vi "Newmark-Test.vi"() -> ()   [LabVIEW 2011]
panel:
  in  "Auto-Catch":bool
  in  "Pre":string
  in  "Post":string
  out "FoyerSonde":i32
  in  "Foyer":i32=5000
  in  "go Sud":bool caption="Ajustement Sud"
  in  "go Ouest":bool caption="Ajustement Est"
  in  "go Nord":bool caption="Ajustement Nord"
  in  "go Est":bool caption="Ajustement Ouest"
  in  "enfoncé":bool
  in  "Foyer+":bool caption="Foyer +"
  in  "Foyer-":bool caption="Foyer -"
  out "X Home":dbl
  in  "Accel":dbl=25000.0
  in  "Fast":dbl=25000.0
  in  "Slow":dbl=10.0
  in  "ActiveStages":string[](array[string])=["AX"]
  out "T Axis":dbl
  out "Z Axis":dbl
  out "Y Axis":dbl
  out "X Axis":dbl
  in  "Auto-Query":bool
  out "In use ?":bool
  in  "CLEAR":bool
  in  "stop":bool
  out "Communication Log":string
  in  "Command String":string
  in  "SendChar":bool
  in  "SendPredefined":bool
  in  "Predefined Commmands":i32(ring) items=["Stop All [SA]", "Referencement", "Home [HM]", "Home Reverse [HR]", "Report Position [PE]", "Status All"]
  in  "Timeout":u32=10000
  in  "baud rate":u32=9600
  in  "VISA resource name":refnum<visa-resource-name>="COM10"
  # "Z"
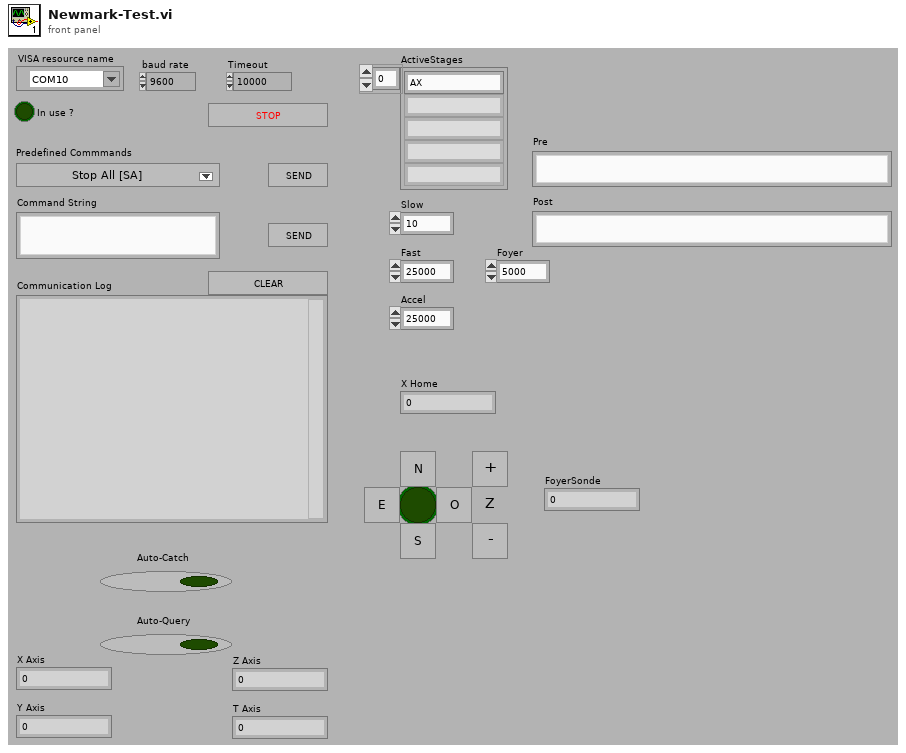
[diagram p1: front panel]
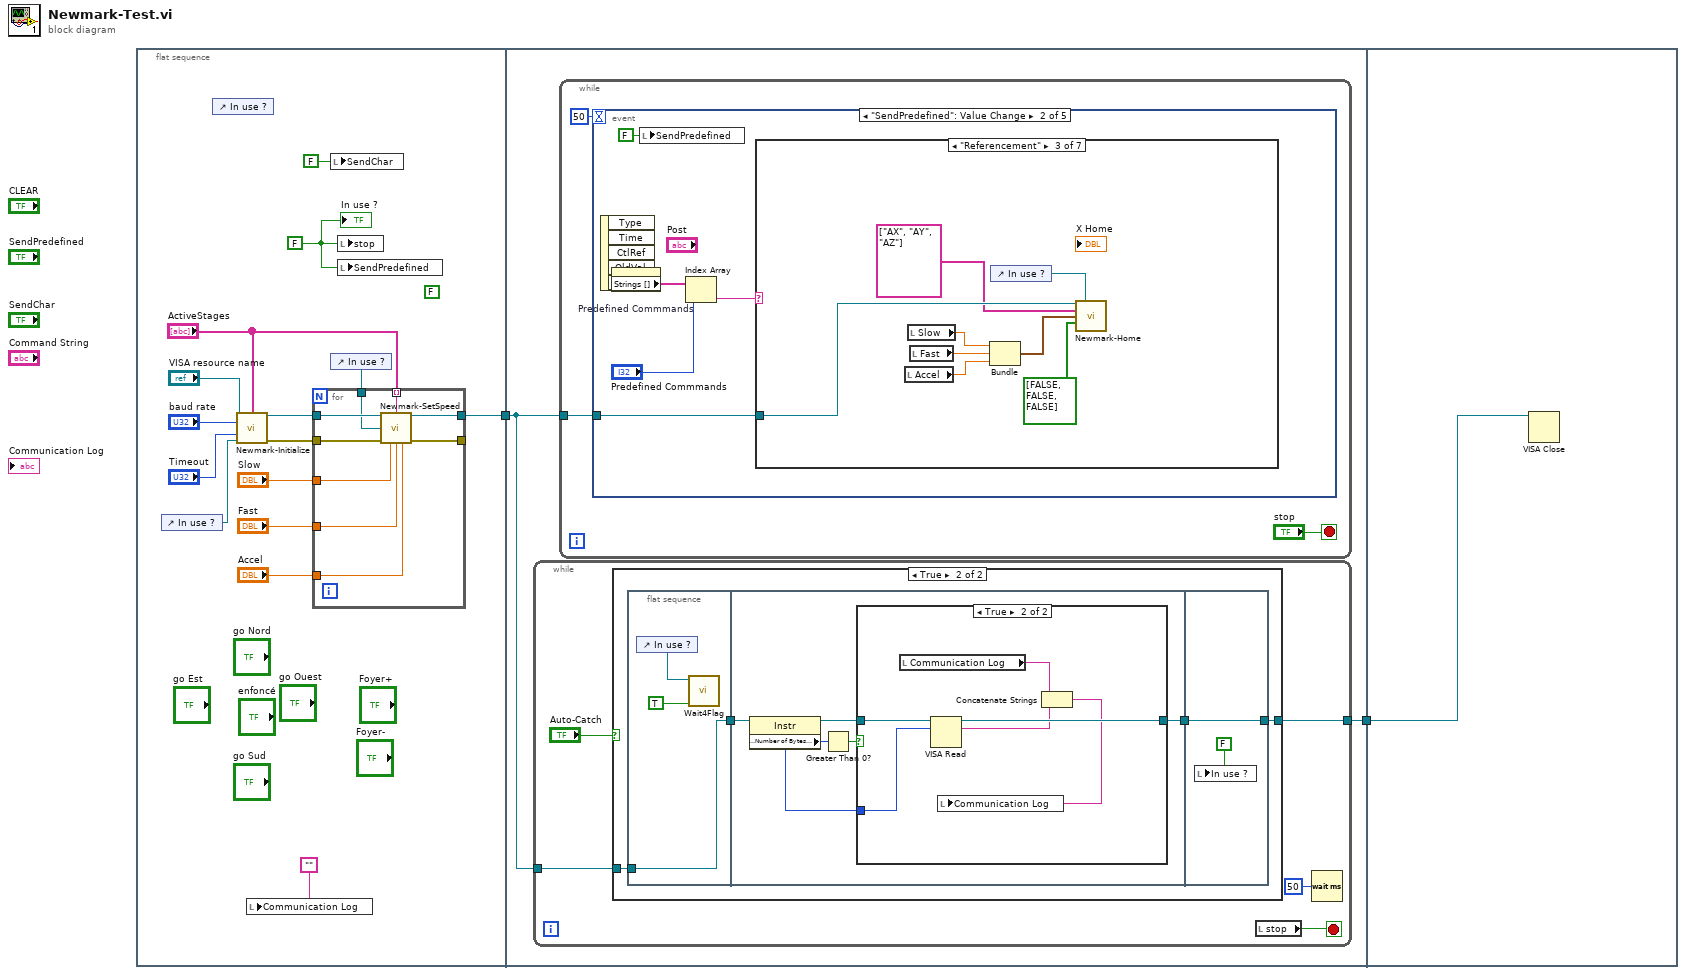
[diagram p0: block diagram]
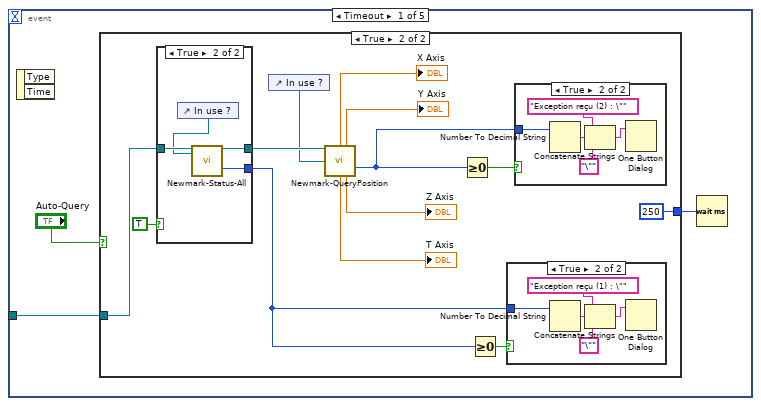
[diagram p4: hidden frame]
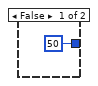
[diagram p5: hidden frame]
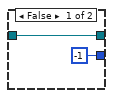
[diagram p6: hidden frame]
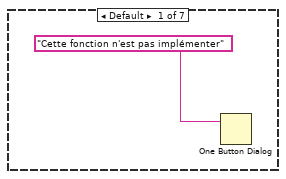
[diagram p9: hidden frame]
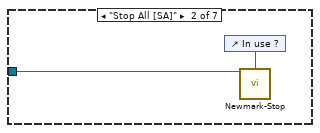
[diagram p10: hidden frame]
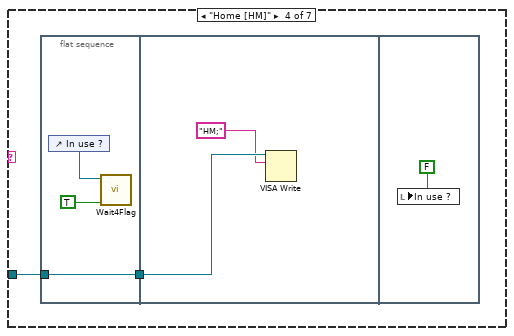
[diagram p11: hidden frame]
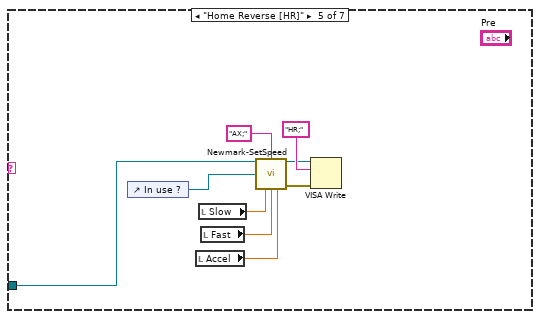
[diagram p12: hidden frame]
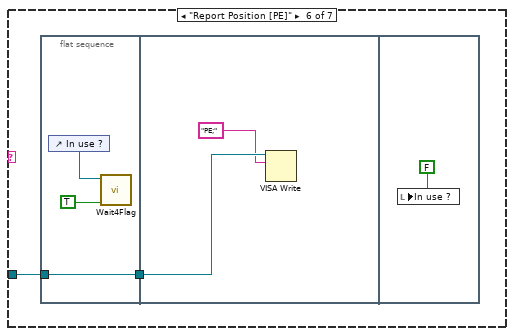
[diagram p13: hidden frame]
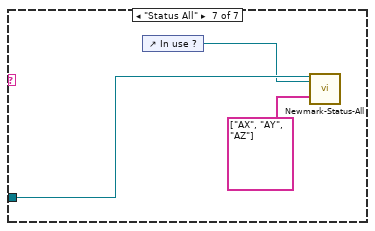
[diagram p14: hidden frame]
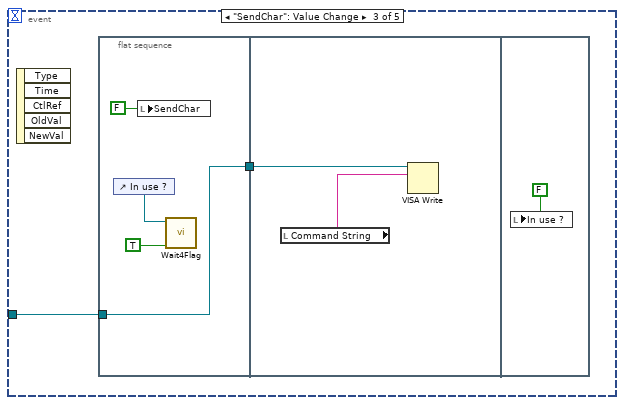
[diagram p15: hidden frame]
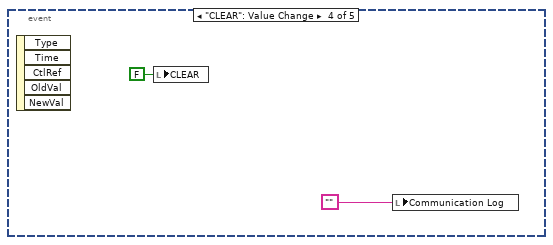
[diagram p16: hidden frame]
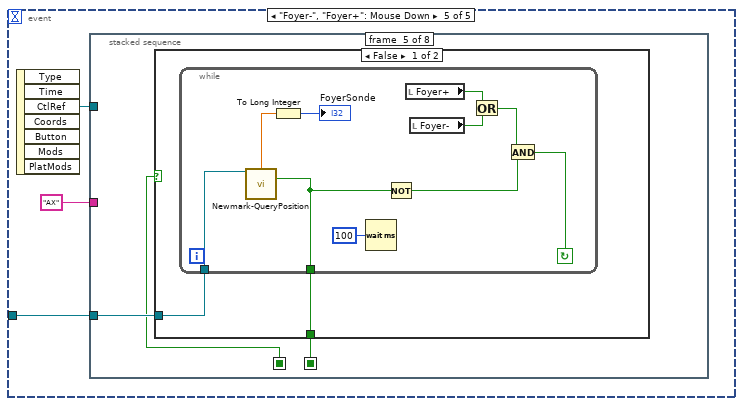
[diagram p17: hidden frame]
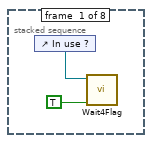
[diagram p18: hidden frame]
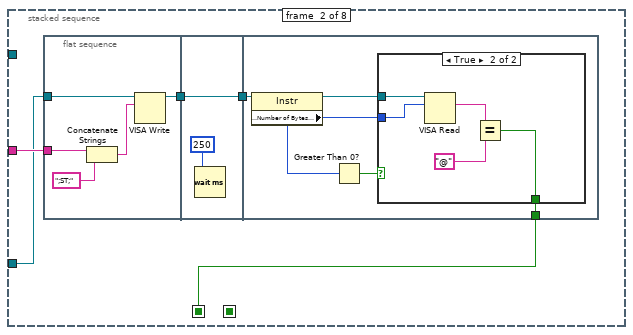
[diagram p19: hidden frame]
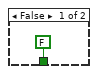
[diagram p20: hidden frame]
diagram:
  n1 = flat-sequence {
    tunnel: [w11] -> w1
    tunnel: [w27] -> w2
    tunnel: w1 -> [w28]
    tunnel: w2 -> [w236]
    frame #0 {
      w16 = FALSE ("Enable Termination\nChar (T)")
      (unwired) FALSE ("Enable Termination\nChar (T)")
      n2 = control-ref of="In use ?"() -> (w3:refnum<vi>)
      n3 = control-ref of="In use ?"() -> ()  [unwired: 1 out]
      n4 = call "Newmark-Initialize.vi"("VISA resource name"="VISA resource name", "ActiveStages"="ActiveStages", "baud rate"="baud rate", "Timeout"="Timeout", "Bool Refnum"=w3) -> ("VISA resource name out"=w10:refnum<visa-resource-name>, "Error OUT"=w8:errorcluster)  [unwired: 8 in, 1 out]
      n5 = local write "Communication Log"("") -> ()
      n6 = local write "SendChar"(FALSE ("Enable Termination\nChar (T)")) -> ()
      n7 = control-ref of="In use ?"() -> (w4:refnum<vi>)
      n8 = for {
        tunnel: w10 -> [w26]
        tunnel: [w25] -> w11
        tunnel: "ActiveStages" -> [w24] mode=indexing
        tunnel: w8 -> [w23]
        tunnel: [w22] -> _
        tunnel: "Slow" -> [w21]
        tunnel: "Fast" -> [w20]
        tunnel: "Accel" -> [w19]
        tunnel: w4 -> [w18]
        n9 = call "Newmark-SetSpeed.vi"("Table VRN"=w26, "StageTAG"=w24, "Bool Refnum"=w18, "Error IN"=w23, "Vitesse Lente"=w21, "Vitesse Rapide"=w20, "Accélération"=w19) -> ("Table VRN OUT"=w25:refnum<visa-resource-name>, "Error OUT"=w22:errorcluster)  [unwired: 6 in, 1 out]
      }
      n10 = local write "stop"(w16) -> ()
      n11 = local write "SendPredefined"(w16) -> ()
      "In use ?" <- w16
    }
    frame #1 {
      n12 = while {
        tunnel: w28 -> [w32]
        tunnel: [w31] -> w27
        stop <- w33 stop-if-true
        n13 = case shown="True" "Auto-Catch" {
          tunnel: w32 -> [w34 w36]
          tunnel: [w34 w35] -> w31
          frame False {
          }
          frame True {
            n14 = flat-sequence {
              tunnel: w36 -> [w41]
              tunnel: [w41] -> w38
              tunnel: w38 -> [w46]
              tunnel: [w43] -> w37
              tunnel: [w55] -> w35
              tunnel: w37 -> [w55]
              frame #0 {
                n15 = control-ref of="In use ?"() -> (w40:refnum<vi>)
                n16 = call "Wait4Flag.vi"("Raise Flag ?"=TRUE, "Ctl Refnum IN"=w40) -> ()  [unwired: 8 in, 2 out]
              }
              frame #1 {
                n17 = property class="Instr"(reference=w46) -> (reference out=w44:refnum<visa-resource-name>, "Serial Settings:Number of Bytes at Serial Port"=w42:u32)  [unwired: 1 in, 1 out]
                n18 = Greater Than 0?(x=w42) -> (x > 0?=w45:bool)
                n19 = case shown="True" w45 {
                  tunnel: w44 -> [w47 w53]
                  tunnel: [w47 w51] -> w43
                  tunnel: w42 -> [_ w52]
                  frame False {
                  }
                  frame True {
                    n20 = local read "Communication Log"() -> (w49:string)
                    n21 = VISA Read(VISA resource name=w53, byte count=w52) -> (VISA resource name out=w51:refnum<visa-resource-name>, read buffer=w50:string)  [unwired: 1 in, 2 out]
                    n22 = Concatenate Strings(w49, w50) -> (w48:string)
                    n23 = local write "Communication Log"(w48) -> ()
                  }
                }
              }
              frame #2 {
                n24 = local write "In use ?"(FALSE ("Enable Termination\nChar (T)")) -> ()
              }
            }
          }
        }
        n25 = local read "stop"() -> (w33:bool)
        n26 = Wait (ms)(milliseconds to wait=u32 50) -> ()  [unwired: 1 out]
      }
      n27 = while {
        tunnel: w28 -> [w57]
        stop <- "stop" stop-if-true
        n28 = event shown="[1] \"SendPredefined\": Value Change" {
          selector: _ -> [_ _ _ _ _]
          dyn-events: _ -> [_ _ _ _ _]
          timeout: 50 -> [_ _ _ _ _]
          tunnel: w57 -> [w61 w92 w137 _ w149]
          event Timeout {
            n29 = event-data() -> ()  [unwired: 1 in, 2 out]
            n30 = case shown="True" "Auto-Query" {
              tunnel: w61 -> [_ w67]
              tunnel: [u32 50 u32 250] -> w59
              frame False {
              }
              frame True {
                n31 = case shown="True" TRUE {
                  tunnel: w67 -> [w77 w81]
                  tunnel: [w77 w80] -> w66
                  tunnel: [-1 ("Exception") w79] -> w65
                  frame False {
                  }
                  frame True {
                    n32 = control-ref of="In use ?"() -> (w78:refnum<vi>)
                    n33 = call "Newmark-Status-All.vi"("Table VRN IN"=w81, "Bool Refnum"=w78) -> ("Table VRN OUT"=w80:refnum<visa-resource-name>, "Exception"=w79:i32)  [unwired: 5 in, 11 out]
                  }
                }
                n34 = control-ref of="In use ?"() -> (w63:refnum<vi>)
                n35 = call "Newmark-QueryPosition.vi"("Table VRN IN"=w66, "Bool Refnum"=w63) -> ("X Axis"=→"X Axis":dbl, "Y Axis"=→"Y Axis":dbl, "Exception"=w71:i32, "T Axis"=→"T Axis":dbl, "Z Axis"=→"Z Axis":dbl)  [unwired: 6 in, 3 out]
                n36 = Greater Or Equal To 0?(x=w71) -> (x >= 0?=w70:bool)
                n37 = Greater Or Equal To 0?(x=w65) -> (x >= 0?=w69:bool)
                n38 = case shown="True" w69 {
                  tunnel: w65 -> [_ w83]
                  frame False {
                  }
                  frame True {
                    n39 = Number To Decimal String(number=w83) -> (decimal integer string=w84:string)  [unwired: 1 in]
                    n40 = Concatenate Strings("Exception reçu (1) : \"" ("string"), w84, "\"" ("string")) -> (w82:string)
                    n41 = One Button Dialog(message=w82) -> ()  [unwired: 1 in, 1 out]
                  }
                }
                n42 = case shown="True" w70 {
                  tunnel: w71 -> [_ w88]
                  frame False {
                  }
                  frame True {
                    n43 = Number To Decimal String(number=w88) -> (decimal integer string=w89:string)  [unwired: 1 in]
                    n44 = Concatenate Strings("Exception reçu (2) : \"" ("string"), w89, "\"" ("string")) -> (w87:string)
                    n45 = One Button Dialog(message=w87) -> ()  [unwired: 1 in, 1 out]
                  }
                }
              }
            }
            n46 = Wait (ms)(milliseconds to wait=w59) -> ()  [unwired: 1 out]
          }
          event "SendPredefined": Value Change {
            n47 = event-data() -> ()  [unwired: 1 in, 5 out]
            n48 = property on="Predefined Commmands" class="Ring (strict)"() -> ("Strings []"=w96:string[])  [unwired: 2 in, 2 out]
            n49 = local write "SendPredefined"(FALSE ("SendPredefined")) -> ()
            n50 = Index Array(array=w96, index="Predefined Commmands") -> (element=w94:string)
            n51 = case shown="\"Referencement\"" w94 {
              tunnel: w92 -> [_ w99 w107 w109 w116 w126 w135]
              frame Default {
                n52 = One Button Dialog(message="Cette fonction n'est pas implémenter") -> ()  [unwired: 1 in, 1 out]
              }
              frame "Stop All [SA]" {
                n53 = control-ref of="In use ?"() -> (w98:refnum<vi>)
                n54 = call "Newmark-Stop.vi"("Table VRN IN"=w99, "Bool Refnum"=w98) -> ()  [unwired: 12 in, 2 out]
              }
              frame "Referencement" {
                n55 = local read "Accel"() -> (w102:dbl)
                n56 = local read "Slow"() -> (w104:dbl)
                n57 = local read "Fast"() -> (w103:dbl)
                n58 = Bundle("Slow"=w104, "Fast"=w103, "Accel"=w102) -> (w101:cluster{"Slow":dbl, "Fast":dbl, "Accel":dbl})  [unwired: 1 in]
                n59 = control-ref of="In use ?"() -> (w100:refnum<vi>)
                n60 = call "Newmark-Home.vi"("Table VRN IN"=w107, "Comm Active"=w100, "StageTAGs"=string[] ["AX", "AY", "AZ"], "Velocities"=w101, "HomeReverse?"=bool[] [FALSE, FALSE, FALSE]) -> ()  [unwired: 9 in, 2 out]
              }
              frame "Home [HM]" {
                n61 = flat-sequence {
                  tunnel: w109 -> [w110]
                  tunnel: [w110] -> w108
                  tunnel: w108 -> [w114]
                  frame #0 {
                    n62 = control-ref of="In use ?"() -> (w111:refnum<vi>)
                    n63 = call "Wait4Flag.vi"("Raise Flag ?"=TRUE, "Ctl Refnum IN"=w111) -> ()  [unwired: 8 in, 2 out]
                  }
                  frame #1 {
                    n64 = VISA Write(VISA resource name=w114, write buffer="HM;") -> ()  [unwired: 1 in, 3 out]
                  }
                  frame #2 {
                    n65 = local write "In use ?"(FALSE ("Enable Termination\nChar (T)")) -> ()
                  }
                }
              }
              frame "Home Reverse [HR]" {
                n66 = control-ref of="In use ?"() -> (w117:refnum<vi>)
                n67 = local read "Accel"() -> (w118:dbl)
                n68 = local read "Slow"() -> (w120:dbl)
                n69 = local read "Fast"() -> (w119:dbl)
                n70 = call "Newmark-SetSpeed.vi"("Table VRN"=w116, "StageTAG"="AX;", "Bool Refnum"=w117, "Vitesse Lente"=w120, "Vitesse Rapide"=w119, "Accélération"=w118) -> ("Table VRN OUT"=w123:refnum<visa-resource-name>, "Error OUT"=w122:errorcluster)  [unwired: 7 in, 1 out]
                n71 = VISA Write(VISA resource name=w123, write buffer="HR;", error in (no error)=w122) -> ()  [unwired: 3 out]
              }
              frame "Report Position [PE]" {
                n72 = flat-sequence {
                  tunnel: w126 -> [w127]
                  tunnel: [w127] -> w125
                  tunnel: w125 -> [w131]
                  frame #0 {
                    n73 = control-ref of="In use ?"() -> (w128:refnum<vi>)
                    n74 = call "Wait4Flag.vi"("Raise Flag ?"=TRUE, "Ctl Refnum IN"=w128) -> ()  [unwired: 8 in, 2 out]
                  }
                  frame #1 {
                    n75 = VISA Write(VISA resource name=w131, write buffer="PE;") -> ()  [unwired: 1 in, 3 out]
                  }
                  frame #2 {
                    n76 = local write "In use ?"(FALSE ("Enable Termination\nChar (T)")) -> ()
                  }
                }
              }
              frame "Status All" {
                n77 = control-ref of="In use ?"() -> (w134:refnum<vi>)
                n78 = call "Newmark-Status-All.vi"("Table VRN IN"=w135, "Bool Refnum"=w134, "StageTag"=string[] ["AX", "AY", "AZ"]) -> ()  [unwired: 4 in, 13 out]
              }
            }
          }
          event "SendChar": Value Change {
            n79 = event-data() -> ()  [unwired: 1 in, 5 out]
            n80 = flat-sequence {
              tunnel: w137 -> [w139]
              tunnel: [w139] -> w136
              tunnel: w136 -> [w143]
              frame #0 {
                n81 = control-ref of="In use ?"() -> (w141:refnum<vi>)
                n82 = local write "SendChar"(FALSE ("Enable Termination\nChar (T)")) -> ()
                n83 = call "Wait4Flag.vi"("Raise Flag ?"=TRUE, "Ctl Refnum IN"=w141) -> ()  [unwired: 8 in, 2 out]
              }
              frame #1 {
                n84 = local read "Command String"() -> (w142:string)
                n85 = VISA Write(VISA resource name=w143, write buffer=w142) -> ()  [unwired: 1 in, 3 out]
              }
              frame #2 {
                n86 = local write "In use ?"(FALSE ("Enable Termination\nChar (T)")) -> ()
              }
            }
          }
          event "CLEAR": Value Change {
            n87 = event-data() -> ()  [unwired: 1 in, 5 out]
            n88 = local write "CLEAR"(FALSE ("CLEAR")) -> ()
            n89 = local write "Communication Log"("") -> ()
          }
          event "Foyer-", "Foyer+": Mouse Down {
            n90 = event-data() -> ("CtlRef"=w147:refnum<vi>)  [unwired: 1 in, 6 out]
            n91 = stacked-sequence {
              seq-local: [_ _ _ _ w200 _ _ _] -> [_ _ _ _ _ w216 _ _]
              seq-local: [_ w152 _ _ _ _ _ _] -> [_ _ w175 w182 w199 w215 w228 _]
              tunnel: w149 -> [_ w155 _ w184 w201 w218 _ _]
              tunnel: "AX" -> [_ w156 w176 w189 _ w217 w229 _]
              tunnel: w147 -> [_ _ _ w195 _ _ _ _]
              frame #0 {
                n92 = control-ref of="In use ?"() -> (w150:refnum<vi>)
                n93 = call "Wait4Flag.vi"("Raise Flag ?"=TRUE, "Ctl Refnum IN"=w150) -> ()  [unwired: 8 in, 2 out]
              }
              frame #1 {
                n94 = flat-sequence {
                  tunnel: w156 -> [w161]
                  tunnel: w155 -> [w158]
                  tunnel: [w157] -> w154
                  tunnel: w154 -> [w163]
                  tunnel: [w163] -> w153
                  tunnel: w153 -> [w168]
                  tunnel: [w164] -> w152
                  frame #0 {
                    n95 = Concatenate Strings(w161, ";ST;") -> (w159:string)
                    n96 = VISA Write(VISA resource name=w158, write buffer=w159) -> (VISA resource name out=w157:refnum<visa-resource-name>)  [unwired: 1 in, 2 out]
                  }
                  frame #1 {
                    n97 = Wait (ms)(milliseconds to wait=u32 250) -> ()  [unwired: 1 out]
                  }
                  frame #2 {
                    n98 = property class="Instr"(reference=w168) -> (reference out=w166:refnum<visa-resource-name>, "Serial Settings:Number of Bytes at Serial Port"=w165:u32)  [unwired: 1 in, 1 out]
                    n99 = Greater Than 0?(x=w165) -> (x > 0?=w167:bool)
                    n100 = case shown="True" w167 {
                      tunnel: w166 -> [_ w174]
                      tunnel: w165 -> [_ w173]
                      tunnel: [FALSE w170] -> w164
                      frame False {
                      }
                      frame True {
                        n101 = VISA Read(VISA resource name=w174, byte count=w173) -> (read buffer=w172:string)  [unwired: 1 in, 3 out]
                        n102 = Equal?(x=w172, y="@") -> (x = y?=w170:bool)
                      }
                    }
                  }
                }
              }
              frame #2 {
                # "Axe du foyer"
                n103 = case shown="False" w175 {
                  tunnel: w176 -> [w178 _]
                  frame False {
                    n104 = local read "Slow"() -> (w179:dbl)
                    n105 = local read "Accel"() -> (w177:dbl)
                    n106 = call "Newmark-SetSpeed.vi"("StageTAG"=w178, "Vitesse Lente"=w179, "Vitesse Rapide"="Foyer", "Accélération"=w177) -> ()  [unwired: 9 in, 3 out]
                  }
                  frame True {
                    n107 = One Button Dialog(message="L'étage du foyer a déjà atteint sa limte de déplacement.") -> ()  [unwired: 1 in, 1 out]
                  }
                }
              }
              frame #3 {
                n108 = property class="Bool (strict)"(reference=w195) -> ("Label.Text"=w194:string)  [unwired: 1 in, 2 out]
                n109 = local read "Foyer"() -> (w196:i32)
                n110 = Equal?(x=w194, y="Foyer+") -> (x = y?=w193:bool)
                n111 = Number To Decimal String(number=w196) -> (decimal integer string=w186:string)  [unwired: 1 in]
                n112 = Select(t="+", s=w193, f="-") -> (s? t:f=w187:string)
                n113 = Concatenate Strings(w189, ";JG", w187, w186, ";") -> (w183:string)
                n114 = case shown="False" w182 {
                  tunnel: w184 -> [w198 _]
                  tunnel: w183 -> [w197 _]
                  frame False {
                    n115 = VISA Write(VISA resource name=w198, write buffer=w197) -> ()  [unwired: 1 in, 3 out]
                  }
                  frame True {
                  }
                }
              }
              frame #4 {
                n116 = case shown="False" w199 {
                  tunnel: w201 -> [w203 _]
                  tunnel: [w202 FALSE ("OverTravel?")] -> w200
                  frame False {
                    n117 = while {
                      tunnel: w203 -> [w210]
                      tunnel: [w204] -> w202
                      stop <- w206 continue-if-true
                      n118 = call "Newmark-QueryPosition.vi"("Table VRN IN"=w210) -> ("X Axis"=w209:dbl, "Error?"=w204:bool)  [unwired: 7 in, 6 out]
                      n119 = To Long Integer(number=w209) -> (32bit integer=→"FoyerSonde":i32)
                      n120 = Wait (ms)(milliseconds to wait=u32 100) -> ()  [unwired: 1 out]
                      n121 = Not(x=w204) -> (.not. x?=w205:bool)
                      n122 = local read "Foyer+"() -> (w213:bool)
                      n123 = local read "Foyer-"() -> (w212:bool)
                      n124 = Or(x=w213, y=w212) -> (x .or. y?=w207:bool)
                      n125 = And(x=w207, y=w205) -> (x .and. y?=w206:bool)
                    }
                  }
                  frame True {
                  }
                }
              }
              frame #5 {
                n126 = case shown="True" w215 {
                  tunnel: w218 -> [w221 _]
                  tunnel: w217 -> [w220 _]
                  tunnel: w216 -> [w219 _]
                  frame False {
                    n127 = case shown="False" w219 {
                      tunnel: w221 -> [w225 _]
                      tunnel: w220 -> [w224 _]
                      frame False {
                        n128 = Concatenate Strings(w224, ";ST;") -> (w222:string)
                        n129 = VISA Write(VISA resource name=w225, write buffer=w222) -> ()  [unwired: 1 in, 3 out]
                      }
                      frame True {
                        n130 = One Button Dialog(message="Le stage de foyer a atteint une limite de déplacement.") -> ()  [unwired: 1 in, 1 out]
                      }
                    }
                  }
                  frame True {
                  }
                }
              }
              frame #6 {
                # "Axe du foyer"
                n131 = control-ref of="In use ?"() -> (w227:refnum<vi>)
                n132 = case shown="False" w228 {
                  tunnel: w229 -> [w234 _]
                  tunnel: w227 -> [w230 _]
                  frame False {
                    n133 = local read "Accel"() -> (w232:dbl)
                    n134 = local read "Slow"() -> (w233:dbl)
                    n135 = local read "Fast"() -> (w231:dbl)
                    n136 = call "Newmark-SetSpeed.vi"("StageTAG"=w234, "Bool Refnum"=w230, "Vitesse Lente"=w233, "Vitesse Rapide"=w231, "Accélération"=w232) -> ()  [unwired: 8 in, 3 out]
                  }
                  frame True {
                  }
                }
              }
              frame #7 {
                n137 = local write "In use ?"(FALSE ("Enable Termination\nChar (T)")) -> ()
              }
            }
          }
        }
      }
    }
    frame #2 {
      n138 = VISA Close(VISA resource name=w236) -> ()  [unwired: 1 in, 1 out]
    }
  }
